vi "Set Message.vi"(8 "error in (no error)":errorcluster, 10 "Message Name":T1, 11 "ATM Controller in":refnum<class "ATM Controller.lvclass">) -> (0 "error out":errorcluster, 3 "ATM Controller out":refnum<class "ATM Controller.lvclass">)   [LabVIEW 2019, in "ATM Controller.lvlib" / "ATM Controller.lvclass"]
uses:
  ATM Controller.lvclass
  Sim Display Console Actor/ATM Controller/Message Name.ctl
  ATM Controller.lvclass/ATM Controller.ctl
  Sim Display Console Actor/Sim Display Console Actor Messages/Write Message Msg/Write Message Msg.lvclass/Write Message Msg.ctl
  <vilib>/ActorFramework/Message Enqueuer/Message Enqueuer.lvclass/Message Enqueuer.ctl
  <vilib>/ActorFramework/Message Enqueuer/Enqueue.vi
  Sim Display Console Actor/Sim Display Console Actor Messages/Write Message Msg/Write Message Msg.lvclass
  C:/Program Files (x86)/National Instruments/LabVIEW 2019/vi.lib/ActorFramework/Message/Message.lvclass
  <vilib>/ActorFramework/Message Priority Queue/Priority Enqueue.vi
  Sim Display Console Actor/ATM Controller/Sim Display Console Actor.lvclass
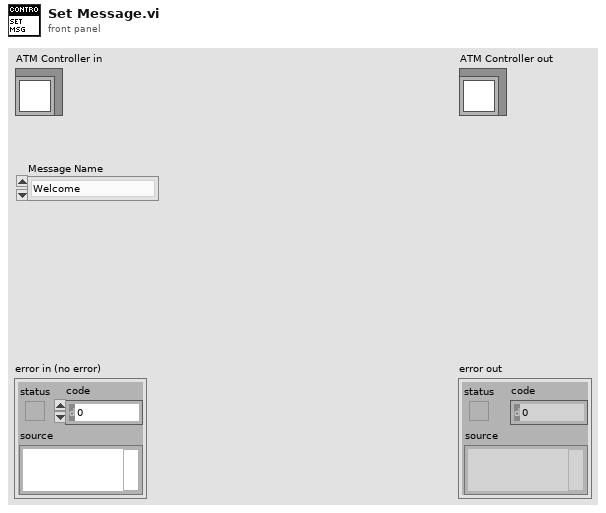
[diagram p1: front panel]
types:
  T1 = typedef "Sim Display Console Actor.lvlib/Sim Display Console Actor.lvclass/Message Name.ctl" = enum16{"Welcome", "Login", "Idle", "Invalid Login", "Terminate Session", "Deposit", "Withdrawal", "Fast Cash $50", "Withdrawal Complete", "Withdrawal Failed", "Balance Inquiry"}
  T2 = typedef "ATM Controller.lvlib/ATM Controller.lvclass/ATM Message.ctl" = string[][]
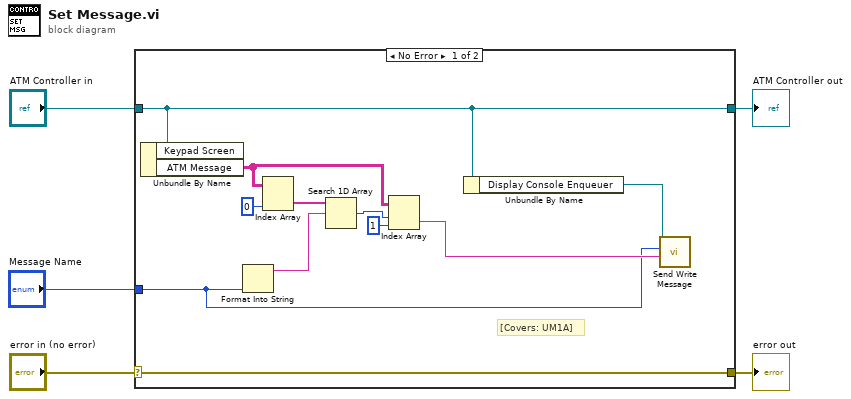
[diagram p0: block diagram]
diagram:
  n1 = case shown="No Error" "error in (no error)" {
    selector: "error in (no error)" -> [w16 w18]
    tunnel: [w16 w18] -> w4
    tunnel: [w13 w17] -> w2
    tunnel: "ATM Controller in" -> [w13 w17]
    tunnel: "Message Name" -> [w6 _]
    frame No Error {
      # "[Covers: UM1A]"
      n2 = Unbundle By Name(w13) -> ("ATM Message"=w12:T2)  [unwired: 1 out]
      n3 = Format Into String(w6) -> (resulting string=w9:string)  [unwired: 3 in, 1 out]
      n4 = Index Array(array=w12, index (col)=0 ("disabled index (col)")) -> (element=w14:string[])  [unwired: 1 in]
      n5 = Search 1D Array(1D array=w14, element=w9) -> (index of element=w8:i32)  [unwired: 1 in]
      n6 = Index Array(array=w12, index (row)=w8, index (col)=1 ("disabled index (col)")) -> (element=w7:string)
      n7 = Unbundle By Name(w13) -> ("Display Console Enqueuer"=w15:refnum<class "Message Enqueuer.lvclass">)
      n8 = call "Send Write Message.vi"("Message Text"=w7, "Message Name"=w6, "Message Enqueuer"=w15) -> ()  [unwired: 7 in, 2 out]
    }
    frame Error {
    }
  }
  "error out" <- w4
  "ATM Controller out" <- w2
